vi "原位（Action).vi"(8 "error in (no error)":errorcluster caption="错误输入（无错误）", 11 "Data In":T1) -> (0 "error out":errorcluster caption="错误输出", 3 "Data Out":T1)   [LabVIEW 2013]
uses:
  Control/Data.ctl
  Control/YV.ctl
  Control/SW.ctl
  Control/State.ctl
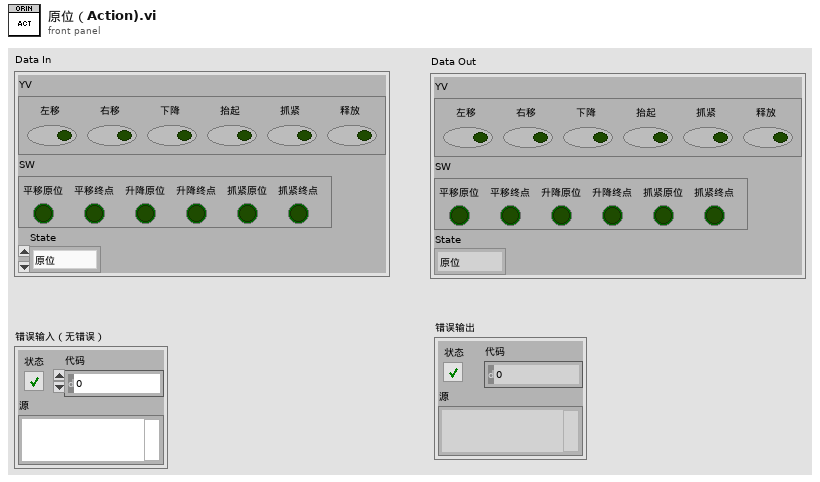
[diagram p1: front panel]
types:
  T1 = typedef "Data.ctl" = cluster{"YV":T2, "SW":T3, "State":T4}
  T2 = typedef "YV.ctl" = cluster{"左移":bool, "右移":bool, "下降":bool, "抬起":bool, "抓紧":bool, "释放":bool}
  T3 = typedef "SW.ctl" = cluster{"平移原位":bool, "平移终点":bool, "升降原位":bool, "升降终点":bool, "抓紧原位":bool, "抓紧终点":bool}
  T4 = typedef "State.ctl" = enum16{"原位", "A侧下降", "夹紧工件", "A侧抬起", "右移", "B侧下降", "释放工件", "B侧抬起", "左移"}
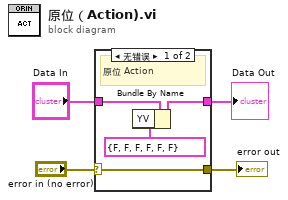
[diagram p0: block diagram]
diagram:
  n1 = case shown="无错误" "error in (no error)" {
    selector: "error in (no error)" -> [w8 w10]
    tunnel: [w8 w10] -> w3
    tunnel: "Data In" -> [w7 w9]
    tunnel: [w6 w9] -> w1
    frame No Error {
      # "原位 Action"
      n2 = Bundle By Name(cluster=w7, "YV"=T2 {"左移"=FALSE, "右移"=FALSE, "下降"=FALSE, "抬起"=FALSE, "抓紧"=FALSE, "释放"=FALSE}) -> (w6:T1)
    }
    frame Error {
    }
  }
  "Data Out" <- w1
  "error out" <- w3
